vi "Matrix Exp.vi"   [LabVIEW 2017, in "NI_AALBase.lvlib"]
doc: "Computes the exponential of a square <B>Input Matrix</B>. Wire data to the <B>Input Matrix</B> input to determine the polymorphic instance to use or manually select the instance."
uses:
  <vilib>/Analysis/NI_AALBase.lvlib
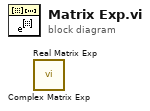
[diagram p0: block diagram]
diagram:
  n1 = call <vilib>:"Complex Matrix Exp.vi"() -> ()  [unwired: 2 in, 2 out]
  n2 = call <vilib>:"Real Matrix Exp.vi"() -> ()  [unwired: 2 in, 2 out]
